vi "Lightning Teleop.vi"(8 "Co_fifo":refnum<k33>, 9 "drive log":refnum<file>, 10 "mechanism log":refnum<file>, 11 "rt fifo":refnum<k33>) -> ()   [LabVIEW 2014]
uses:
  TeleopCmd.ctl
  CmdFlag.ctl
  Co-Pilot_game_control.ctl
  <vilib>/Rock Robotics/WPI/Joystick/WPI_JoystickGetSetRefNum.vi
  <vilib>/Rock Robotics/Network Tables/SD Read Boolean.vi
panel:
  out "Axes":dbl[](array[numeric])
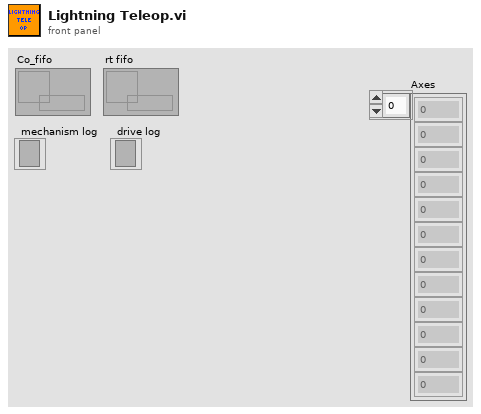
[diagram p1: front panel]
types:
  T1 = typedef "CmdFlag.ctl" = enum16{"noop", "logflag", "suspend", "resume"}
  T2 = typedef "Co-Pilot_game_control.ctl" = cluster{"Left_Intake":dbl, "Right_Intake":dbl, "Time Stamp":u32, "Command":enum16{"Noop", "Flagged"}, "ToggleCollector":bool, "ManualLift":dbl, "Top_Limit_Switch":bool, "Bottom_Limit_Switch ":bool, "LifterOverride":bool, "AutoLift":i32, "Toggle Auto Lifter":bool, "Activate HP indexer":bool}
  T3 = typedef "TeleopCmd.ctl" = cluster{"CmdFlag":T1, "throttle":dbl, "turn":dbl, "Override":bool, "Strafe":dbl, "MotorPwrMax":u8, "Time":u32, "ultrasonic override":bool}
  T4 = typedef "WPI_JoystickDevRef.ctl" = cluster{"Device":T5}
  T5 = typedef "WPI_JoystickDeviceEnum.ctl" = enum16{"USB 0", "USB 1", "USB 2", "USB 3", "USB 4", "USB 5"}
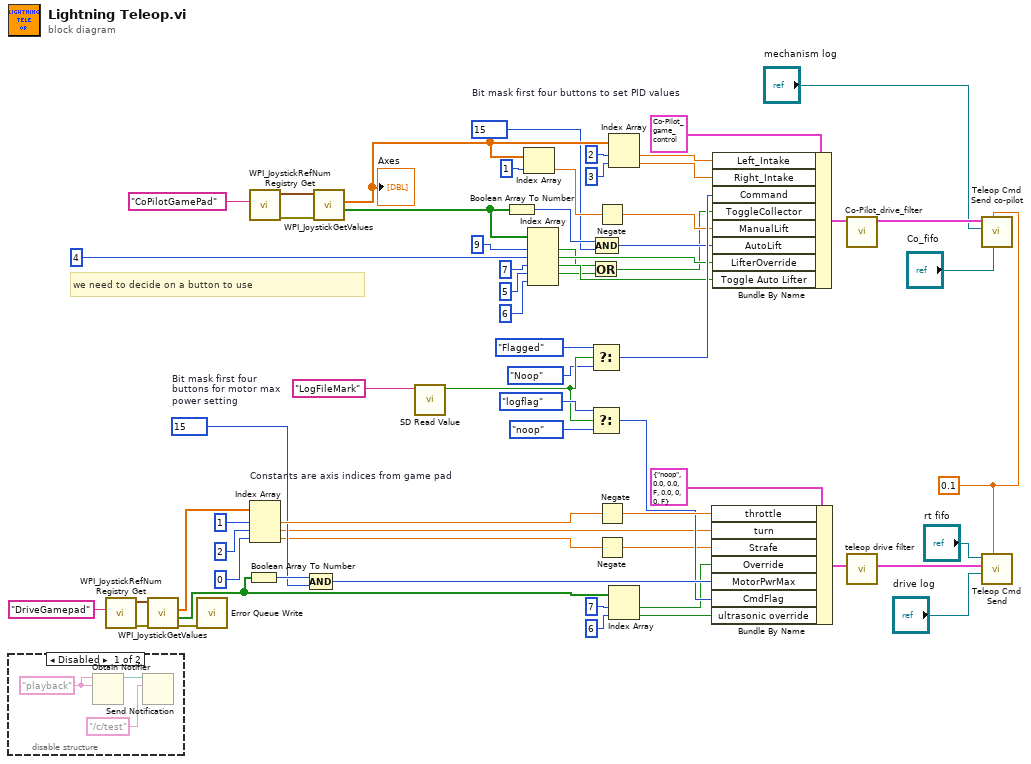
[diagram p0: block diagram]
diagram:
  w1 = 0.1 ("Epsilon")
  w11 = u32 15  # Bit mask first four buttons to set PID values
  w52 = u32 15  # Bit mask first four buttons for motor max power setting
  # "we need to decide on a button to use"
  n1 = disable-structure shown="Disabled" {
    frame Disabled {
      w67 = "playback" ("name (unnamed)")
      n2 = Obtain Notifier(name (unnamed)=w67, notification data type=w67) -> (notifier out=w68:refnum<notifier>)  [unwired: 2 in, 2 out]
      n3 = Send Notification(notification="/c/test", notifier=w68) -> ()  [unwired: 1 in, 2 out]
    }
    frame Enabled {
    }
  }
  n4 = call <vilib>:"WPI_JoystickRefNum Registry Get.vi"("refnum name"="DriveGamepad") -> ("error out"=w50:errorcluster, "JoystickDevRef"=w61:T4)  [unwired: 9 in]
  n5 = call <vilib>:"WPI_JoystickGetValues.vi"("error in (no error)"=w50, "JoystickDevRef"=w61) -> ("error out"=w49:errorcluster, "Buttons"=w54:bool[], "Axes"=w60:dbl[])  [unwired: 5 in, 2 out]
  n6 = call "Error Queue Write.vi"("error in (no error)"=w49) -> ()  [unwired: 11 in]
  n7 = Boolean Array To Number(Boolean array=w54) -> (number=w53:u32)
  n8 = call <vilib>:"WPI_JoystickRefNum Registry Get.vi"("refnum name"="CoPilotGamePad") -> ("error out"=w46:errorcluster, "JoystickDevRef"=w45:T4)  [unwired: 9 in]
  n9 = Index Array "Constants are axis indices from game pad"(array=w60, index #1=1 ("index"), index #2=2 ("index"), index #3=0 ("index")) -> (element #1=w56:dbl, element #2=w19:dbl, element #3=w21:dbl)
  n10 = Compound Arithmetic op=AND(w53, w52) -> (w51:u32)
  n11 = call <vilib>:"WPI_JoystickGetValues.vi"("error in (no error)"=w46, "JoystickDevRef"=w45) -> ("Buttons"=w18:bool[], "Axes"=w14:dbl[])  [unwired: 5 in, 3 out]
  "Axes" <- w14
  n12 = call-poly <vilib>:"SD Read Value.vi"("Name"="LogFileMark") -> ("Boolean"=w30:bool)  [unwired: 8 in, 2 out]
  n13 = Boolean Array To Number(Boolean array=w18) -> (number=w12:u32)
  n14 = Index Array(array=w14, index=1) -> (element=w15:dbl)
  n15 = Index Array(array=w18, index #1=9 ("index"), index #2=4 ("index"), index #3=7 ("index"), index #4=5 ("index"), index #5=6 ("index")) -> (element #1=w6:bool, element #2=w9:bool, element #3=w7:bool, element #4=w4:bool)  [unwired: 1 out]
  n16 = Or(x=w6, y=w4) -> (x .or. y?=w3:bool)
  n17 = Select(t=enum16{"Noop", "Flagged"}."Flagged" ("Command"), s=w30, f=enum16{"Noop", "Flagged"}."Noop" ("Command")) -> (s? t:f=w27:enum16{"Noop", "Flagged"})
  n18 = Select(t=CmdFlag."logflag" ("CmdFlag"), s=w30, f=CmdFlag."noop" ("CmdFlag")) -> (s? t:f=w31:T1)
  n19 = Compound Arithmetic op=AND(w12, w11) -> (w10:u32)
  n20 = Negate(x=w15) -> (-x=w13:dbl)
  n21 = Negate(x=w56) -> (-x=w48:dbl)
  n22 = Negate(x=w21) -> (-x=w20:dbl)
  n23 = Index Array(array=w14, index #1=2 ("index"), index #2=3 ("index")) -> (element #1=w42:dbl, element #2=w41:dbl)
  n24 = Index Array(array=w54, index #1=7 ("index"), index #2=6 ("index")) -> (element #1=w24:bool, element #2=w22:bool)
  n25 = Bundle By Name(cluster=T3 {"CmdFlag"=enum."noop", "throttle"=0.0, "turn"=0.0, "Override"=FALSE, "Strafe"=0.0, "MotorPwrMax"=0, "Time"=0, "ultrasonic override"=FALSE} ("Cluster"), "throttle"=w48, "turn"=w19, "Strafe"=w20, "Override"=w24, "MotorPwrMax"=w51, "CmdFlag"=w31, "ultrasonic override"=w22) -> (w64:T3)
  n26 = Bundle By Name(cluster=T2 {"Left_Intake"=0.0, "Right_Intake"=0.0, "Time Stamp"=0, "Command"=enum."Noop", "ToggleCollector"=FALSE, "ManualLift"=0.0, "Top_Limit_Switch"=FALSE, "Bottom_Limit_Switch "=FALSE, "LifterOverride"=FALSE, "AutoLift"=0, "Toggle Auto Lifter"=FALSE, "Activate HP indexer"=FALSE} ("Co-Pilot Data"), "Left_Intake"=w42, "Right_Intake"=w41, "Command"=w27, "ToggleCollector"=w3, "ManualLift"=w13, "AutoLift"=w10, "LifterOverride"=w9, "Toggle Auto Lifter"=w7) -> (w40:T2)
  n27 = call "Co-Pilot_drive_filter.vi"("Co-Pilot Data"=w40) -> ("output cluster"=w39:T2)  [unwired: 10 in]
  n28 = call "teleop drive filter.vi"("input data"=w64) -> ("output data"=w63:T3)  [unwired: 10 in]
  n29 = call "Teleop Cmd Send co-pilot.vi"("Co_fifo"="Co_fifo", "Epsilon"=w1, "mechanism log"="mechanism log", "Co-Pilot Data"=w39) -> ()  [unwired: 7 in, 1 out]
  n30 = call "Teleop Cmd Send.vi"("rt fifo"="rt fifo", "Teleop Inputs"=w63, "drive log"="drive log", "Epsilon"=w1) -> ()  [unwired: 6 in, 1 out]
